vi "4 Wheel Integration.vi"() -> ()   [LabVIEW 2017]
uses:
  <vilib>/robotics/Steering/Wheel/Wheel Parameters.ctl
  <vilib>/robotics/Steering/Wheel/Rotation Direction.ctl
  <vilib>/robotics/Steering/Fixed Wheel/NI_Robotics_Fixed Wheel.lvclass
  C:/Program Files (x86)/National Instruments/LabVIEW 2017/vi.lib/robotics/Steering/Wheel/NI_Robotics_Wheel.lvclass
  <vilib>/robotics/Steering/Fixed Wheel/Create Fixed Wheel.vi
  <vilib>/robotics/Steering/Steering Frame/Create User Defined Steering Frame.vi
  <vilib>/robotics/Steering/Steering Frame/Apply Steering Frame Velocity to Motors.vi
  <vilib>/robotics/Steering/Steering Frame/Get Steering Frame Velocity from Motors.vi
  <vilib>/robotics/Steering/Create Steering Frame/NI_Robotics_Create Steering Frame.xnode
  <vilib>/robotics/Steering/Class Type Definitions/Steering Frame.ctl
  <vilib>/robotics/Steering/Steering Frame/NI_Robotics_Steering Frame.lvclass
  <vilib>/robotics/Steering/Class Type Definitions/NI_Robotics_Steering Class Types.lvlib
  <vilib>/robotics/Steering/Wheel/NI_Robotics_Wheel.lvclass
panel:
  out "estimated steering frame velocity":dbl[](array[numeric])
  out "ccw motor velocity setpoints":dbl[](array[numeric])
  in  "steering frame velocity":dbl[](array[numeric])=[0.0, 0.0, 0.0]
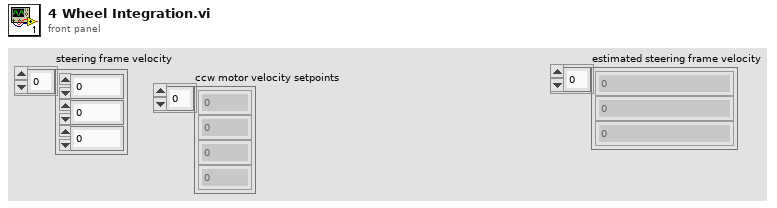
[diagram p1: front panel]
types:
  T1 = typedef "NI_Robotics_Steering Class Types.lvlib/Steering Frame.ctl" = refnum<class "NI_Robotics_Steering Frame.lvclass">
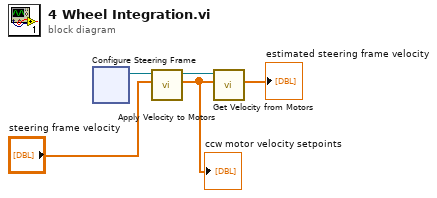
[diagram p0: block diagram]
diagram:
  n1 = xnode ("Configure Steering Frame")() -> ("steering frame out"=w4:T1)  [unwired: 1 in, 1 out]
  n2 = call-poly <vilib>:"Apply Velocity to Motors.vi"("steering frame velocity"="steering frame velocity", "steering frame in"=w4) -> ("ccw motor velocity setpoints"=w1:dbl[], "steering frame out"=w2:T1)  [unwired: 5 in, 3 out]
  "ccw motor velocity setpoints" <- w1
  n3 = call-poly <vilib>:"Get Velocity from Motors.vi"("ccw motor velocity states"=w1, "steering frame in"=w2) -> ("estimated steering frame velocity"=→"estimated steering frame velocity":dbl[])  [unwired: 7 in, 2 out]
